vi "MC - Get Data From Key Value.vi"(0 "Key Value":string[][](array[string])) -> (1 "Date":string[](array[string]), 2 "Interval in Days":string[](array[string]), 3 "Message":string[](array[string]))   [LabVIEW 2015]
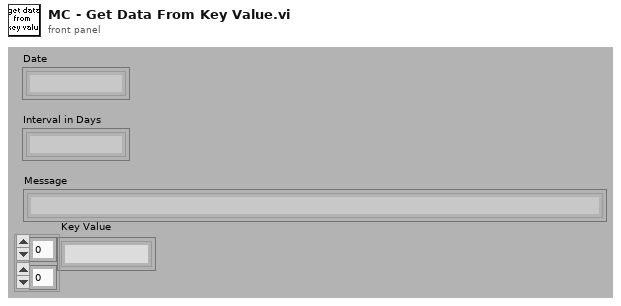
[diagram p1: front panel]
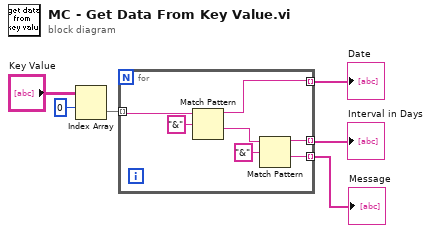
[diagram p0: block diagram]
diagram:
  n1 = Index Array(array="Key Value", index (row)=0) -> (element=w1:string[])  [unwired: 1 in]
  n2 = for {
    tunnel: w1 -> [w10] mode=indexing
    tunnel: [w9] -> w4 mode=indexing
    tunnel: [w8] -> w5 mode=indexing
    tunnel: [w7] -> w6 mode=indexing
    n3 = Match Pattern(string=w10, regular expression="&") -> (before substring=w9:string, after substring=w13:string)  [unwired: 3 out]
    n4 = Match Pattern(string=w13, regular expression="&") -> (before substring=w8:string, after substring=w7:string)  [unwired: 3 out]
  }
  "Date" <- w4
  "Interval in Days" <- w5
  "Message" <- w6
